vi "Line ovelay one.vi"(4 "Thickness":i32, 6 "Group":string, 7 "Color":u32(colorbox)=16711680, 8 "error in (no error)":errorcluster, 9 "End Point":cluster{"X":i32, "Y":i32}, 10 "Start Point":cluster{"X":i32, "Y":i32}, 11 "Image":T1) -> (0 "error out":errorcluster, 3 "Image Out":T1)   [LabVIEW 2015]
uses:
  <vilib>/vision/Image Controls.llb/IMAQ Image.ctl
  nivision.dll
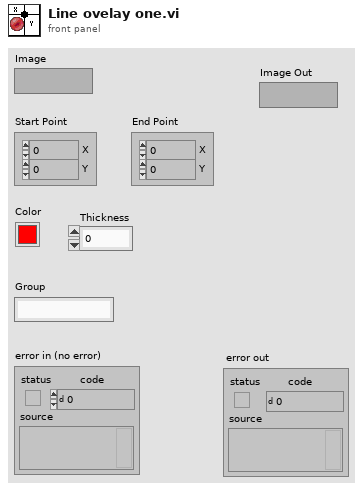
[diagram p1: front panel]
types:
  T1 = typedef "IMAQ Image.ctl" = refnum<image>
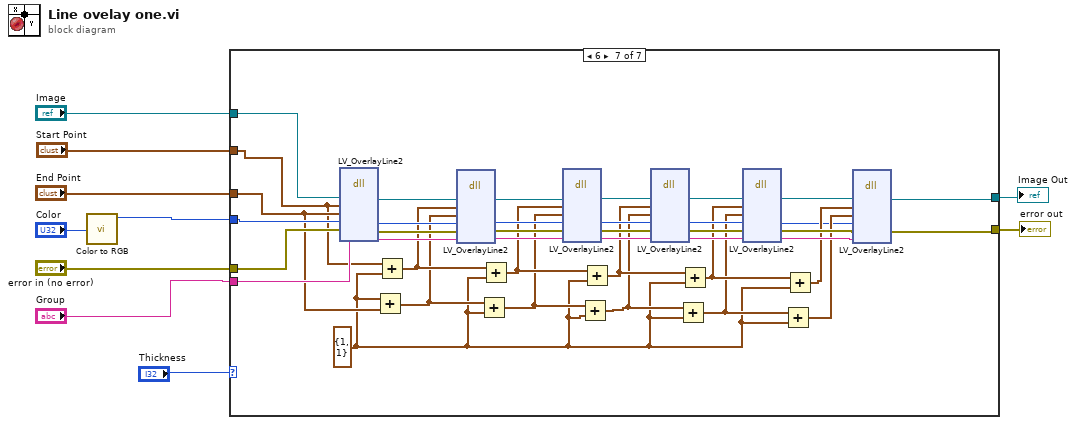
[diagram p0: block diagram]
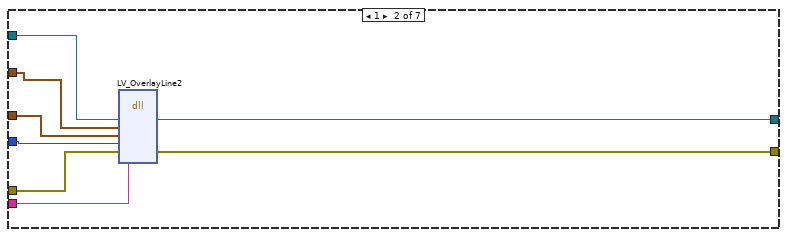
[diagram p3: hidden frame]
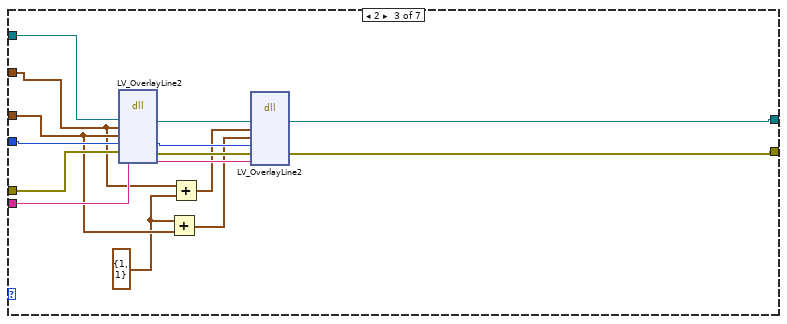
[diagram p4: hidden frame]
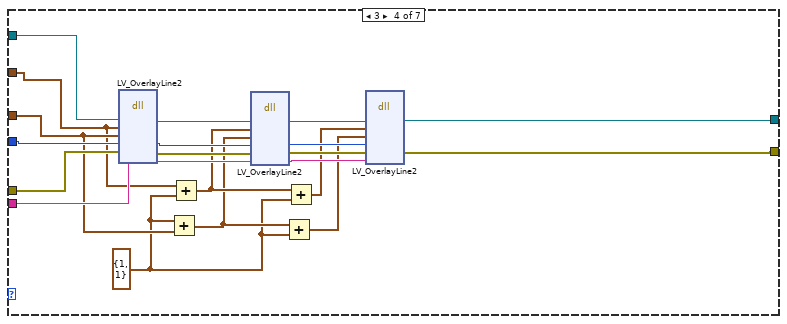
[diagram p5: hidden frame]
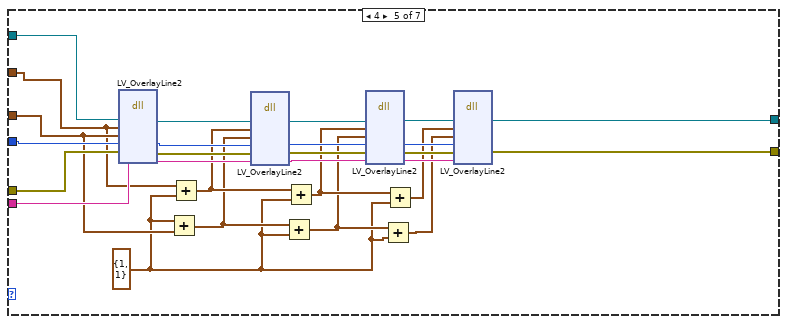
[diagram p6: hidden frame]
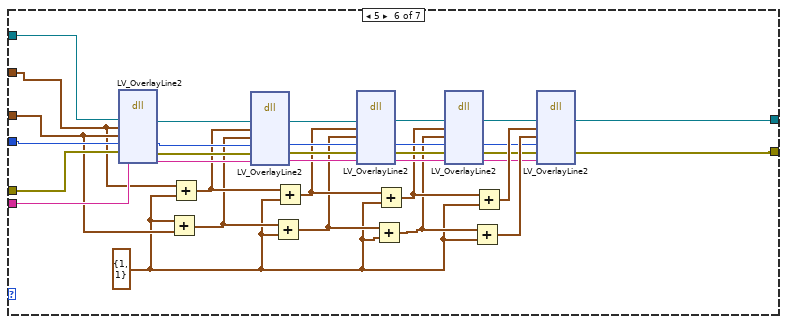
[diagram p7: hidden frame]
diagram:
  n1 = call <vilib>:"Color to RGB.vi"("Color"="Color") -> ("Resolved Color"=w6:u32)  [unwired: 3 out]
  n2 = case shown="6" "Thickness" {
    tunnel: "Group" -> [_ w20 w35 w56 w83 w116 w155]
    tunnel: "error in (no error)" -> [w11 w15 w32 w53 w80 w113 w152]
    tunnel: w6 -> [_ w16 w33 w54 w81 w114 w153]
    tunnel: "End Point" -> [_ w17 w27 w48 w75 w108 w147]
    tunnel: "Start Point" -> [_ w18 w26 w47 w74 w107 w146]
    tunnel: "Image" -> [w12 w19 w34 w55 w82 w115 w154]
    tunnel: [w12 w14 w22 w36 w58 w85 w123] -> w1
    tunnel: [w11 w13 w21 w37 w57 w84 w125] -> w2
    frame 0, Default {
    }
    frame 1 {
      n3 = dll-call lib="nivision.*" fn="LV_OverlayLine2"("src"=w19, "startPoint"=w18, "endPoint"=w17, "color"=w16, "err"=w15, "group"=w20) -> ("src"=w14:T1, "err"=w13:errorcluster)  [unwired: 7 in, 3 out]
    }
    frame 2 {
      w23 = cluster{"X":i32, "Y":i32} {"X"=1, "Y"=1} ("x")
      n4 = dll-call lib="nivision.*" fn="LV_OverlayLine2"("src"=w34, "startPoint"=w26, "endPoint"=w27, "color"=w33, "err"=w32, "group"=w35) -> ("src"=w31:T1, "color"=w28:u32, "err"=w29:errorcluster, "group"=w30:string)  [unwired: 5 in, 3 out]
      n5 = Add(x=w23, y=w27) -> (x+y=w24:cluster{"X":i32, "Y":i32})
      n6 = Add(x=w26, y=w23) -> (x+y=w25:cluster{"X":i32, "Y":i32})
      n7 = dll-call lib="nivision.*" fn="LV_OverlayLine2"("src"=w31, "startPoint"=w25, "endPoint"=w24, "color"=w28, "err"=w29, "group"=w30) -> ("src"=w22:T1, "err"=w21:errorcluster)  [unwired: 7 in, 3 out]
    }
    frame 3 {
      w38 = cluster{"X":i32, "Y":i32} {"X"=1, "Y"=1} ("x")
      n8 = dll-call lib="nivision.*" fn="LV_OverlayLine2"("src"=w55, "startPoint"=w47, "endPoint"=w48, "color"=w54, "err"=w53, "group"=w56) -> ("src"=w52:T1, "color"=w49:u32, "err"=w50:errorcluster, "group"=w51:string)  [unwired: 5 in, 3 out]
      n9 = Add(x=w38, y=w48) -> (x+y=w41:cluster{"X":i32, "Y":i32})
      n10 = Add(x=w47, y=w38) -> (x+y=w42:cluster{"X":i32, "Y":i32})
      n11 = dll-call lib="nivision.*" fn="LV_OverlayLine2"("src"=w52, "startPoint"=w42, "endPoint"=w41, "color"=w49, "err"=w50, "group"=w51) -> ("src"=w46:T1, "color"=w43:u32, "err"=w44:errorcluster, "group"=w45:string)  [unwired: 5 in, 3 out]
      n12 = Add(x=w41, y=w38) -> (x+y=w39:cluster{"X":i32, "Y":i32})
      n13 = Add(x=w42, y=w38) -> (x+y=w40:cluster{"X":i32, "Y":i32})
      n14 = dll-call lib="nivision.*" fn="LV_OverlayLine2"("src"=w46, "startPoint"=w40, "endPoint"=w39, "color"=w43, "err"=w44, "group"=w45) -> ("src"=w36:T1, "err"=w37:errorcluster)  [unwired: 7 in, 3 out]
    }
    frame 4 {
      w59 = cluster{"X":i32, "Y":i32} {"X"=1, "Y"=1} ("x")
      n15 = dll-call lib="nivision.*" fn="LV_OverlayLine2"("src"=w82, "startPoint"=w74, "endPoint"=w75, "color"=w81, "err"=w80, "group"=w83) -> ("src"=w79:T1, "color"=w76:u32, "err"=w77:errorcluster, "group"=w78:string)  [unwired: 5 in, 3 out]
      n16 = Add(x=w59, y=w75) -> (x+y=w68:cluster{"X":i32, "Y":i32})
      n17 = Add(x=w74, y=w59) -> (x+y=w69:cluster{"X":i32, "Y":i32})
      n18 = dll-call lib="nivision.*" fn="LV_OverlayLine2"("src"=w79, "startPoint"=w69, "endPoint"=w68, "color"=w76, "err"=w77, "group"=w78) -> ("src"=w73:T1, "color"=w70:u32, "err"=w71:errorcluster, "group"=w72:string)  [unwired: 5 in, 3 out]
      n19 = Add(x=w68, y=w59) -> (x+y=w62:cluster{"X":i32, "Y":i32})
      n20 = Add(x=w69, y=w59) -> (x+y=w63:cluster{"X":i32, "Y":i32})
      n21 = dll-call lib="nivision.*" fn="LV_OverlayLine2"("src"=w73, "startPoint"=w63, "endPoint"=w62, "color"=w70, "err"=w71, "group"=w72) -> ("src"=w64:T1, "color"=w65:u32, "err"=w66:errorcluster, "group"=w67:string)  [unwired: 5 in, 3 out]
      n22 = Add(x=w62, y=w59) -> (x+y=w60:cluster{"X":i32, "Y":i32})
      n23 = Add(x=w63, y=w59) -> (x+y=w61:cluster{"X":i32, "Y":i32})
      n24 = dll-call lib="nivision.*" fn="LV_OverlayLine2"("src"=w64, "startPoint"=w61, "endPoint"=w60, "color"=w65, "err"=w66, "group"=w67) -> ("src"=w58:T1, "err"=w57:errorcluster)  [unwired: 7 in, 3 out]
    }
    frame 5 {
      w92 = cluster{"X":i32, "Y":i32} {"X"=1, "Y"=1} ("x")
      n25 = dll-call lib="nivision.*" fn="LV_OverlayLine2"("src"=w115, "startPoint"=w107, "endPoint"=w108, "color"=w114, "err"=w113, "group"=w116) -> ("src"=w112:T1, "color"=w109:u32, "err"=w110:errorcluster, "group"=w111:string)  [unwired: 5 in, 3 out]
      n26 = Add(x=w92, y=w108) -> (x+y=w101:cluster{"X":i32, "Y":i32})
      n27 = Add(x=w107, y=w92) -> (x+y=w102:cluster{"X":i32, "Y":i32})
      n28 = dll-call lib="nivision.*" fn="LV_OverlayLine2"("src"=w112, "startPoint"=w102, "endPoint"=w101, "color"=w109, "err"=w110, "group"=w111) -> ("src"=w106:T1, "color"=w103:u32, "err"=w104:errorcluster, "group"=w105:string)  [unwired: 5 in, 3 out]
      n29 = Add(x=w101, y=w92) -> (x+y=w95:cluster{"X":i32, "Y":i32})
      n30 = Add(x=w102, y=w92) -> (x+y=w96:cluster{"X":i32, "Y":i32})
      n31 = dll-call lib="nivision.*" fn="LV_OverlayLine2"("src"=w106, "startPoint"=w96, "endPoint"=w95, "color"=w103, "err"=w104, "group"=w105) -> ("src"=w97:T1, "color"=w98:u32, "err"=w99:errorcluster, "group"=w100:string)  [unwired: 5 in, 3 out]
      n32 = Add(x=w95, y=w92) -> (x+y=w93:cluster{"X":i32, "Y":i32})
      n33 = Add(x=w96, y=w92) -> (x+y=w94:cluster{"X":i32, "Y":i32})
      n34 = dll-call lib="nivision.*" fn="LV_OverlayLine2"("src"=w97, "startPoint"=w94, "endPoint"=w93, "color"=w98, "err"=w99, "group"=w100) -> ("src"=w86:T1, "color"=w87:u32, "err"=w88:errorcluster, "group"=w89:string)  [unwired: 5 in, 3 out]
      n35 = Add(x=w93, y=w92) -> (x+y=w90:cluster{"X":i32, "Y":i32})
      n36 = Add(x=w94, y=w92) -> (x+y=w91:cluster{"X":i32, "Y":i32})
      n37 = dll-call lib="nivision.*" fn="LV_OverlayLine2"("src"=w86, "startPoint"=w91, "endPoint"=w90, "color"=w87, "err"=w88, "group"=w89) -> ("src"=w85:T1, "err"=w84:errorcluster)  [unwired: 7 in, 3 out]
    }
    frame 6 {
      w120 = cluster{"X":i32, "Y":i32} {"X"=1, "Y"=1} ("x")
      n38 = dll-call lib="nivision.*" fn="LV_OverlayLine2"("src"=w154, "startPoint"=w146, "endPoint"=w147, "color"=w153, "err"=w152, "group"=w155) -> ("src"=w151:T1, "color"=w148:u32, "err"=w149:errorcluster, "group"=w150:string)  [unwired: 5 in, 3 out]
      n39 = Add(x=w120, y=w147) -> (x+y=w140:cluster{"X":i32, "Y":i32})
      n40 = Add(x=w146, y=w120) -> (x+y=w141:cluster{"X":i32, "Y":i32})
      n41 = dll-call lib="nivision.*" fn="LV_OverlayLine2"("src"=w151, "startPoint"=w141, "endPoint"=w140, "color"=w148, "err"=w149, "group"=w150) -> ("src"=w145:T1, "color"=w142:u32, "err"=w143:errorcluster, "group"=w144:string)  [unwired: 5 in, 3 out]
      n42 = Add(x=w140, y=w120) -> (x+y=w134:cluster{"X":i32, "Y":i32})
      n43 = Add(x=w141, y=w120) -> (x+y=w135:cluster{"X":i32, "Y":i32})
      n44 = dll-call lib="nivision.*" fn="LV_OverlayLine2"("src"=w145, "startPoint"=w135, "endPoint"=w134, "color"=w142, "err"=w143, "group"=w144) -> ("src"=w136:T1, "color"=w137:u32, "err"=w138:errorcluster, "group"=w139:string)  [unwired: 5 in, 3 out]
      n45 = Add(x=w134, y=w120) -> (x+y=w132:cluster{"X":i32, "Y":i32})
      n46 = Add(x=w135, y=w120) -> (x+y=w133:cluster{"X":i32, "Y":i32})
      n47 = dll-call lib="nivision.*" fn="LV_OverlayLine2"("src"=w136, "startPoint"=w133, "endPoint"=w132, "color"=w137, "err"=w138, "group"=w139) -> ("src"=w128:T1, "color"=w129:u32, "err"=w130:errorcluster, "group"=w131:string)  [unwired: 5 in, 3 out]
      n48 = Add(x=w132, y=w120) -> (x+y=w121:cluster{"X":i32, "Y":i32})
      n49 = Add(x=w133, y=w120) -> (x+y=w122:cluster{"X":i32, "Y":i32})
      n50 = dll-call lib="nivision.*" fn="LV_OverlayLine2"("src"=w128, "startPoint"=w122, "endPoint"=w121, "color"=w129, "err"=w130, "group"=w131) -> ("src"=w124:T1, "color"=w117:u32, "err"=w126:errorcluster, "group"=w127:string)  [unwired: 5 in, 3 out]
      n51 = Add(x=w121, y=w120) -> (x+y=w118:cluster{"X":i32, "Y":i32})
      n52 = Add(x=w122, y=w120) -> (x+y=w119:cluster{"X":i32, "Y":i32})
      n53 = dll-call lib="nivision.*" fn="LV_OverlayLine2"("src"=w124, "startPoint"=w119, "endPoint"=w118, "color"=w117, "err"=w126, "group"=w127) -> ("src"=w123:T1, "err"=w125:errorcluster)  [unwired: 7 in, 3 out]
    }
  }
  "Image Out" <- w1
  "error out" <- w2
